vi "Get All.vi"(7 "Q Ref In":refnum<queue>, 8 "error in":errorcluster) -> (0 "error out":errorcluster, 3 "Flushed Elements":T1[](array[typedef]), 5 "Q Ref Out":refnum<queue>)   [LabVIEW 2025, in "Q Wrappers.lvlib"]
uses:
  Q Wrappers.lvlib
  Q Packet.ctl
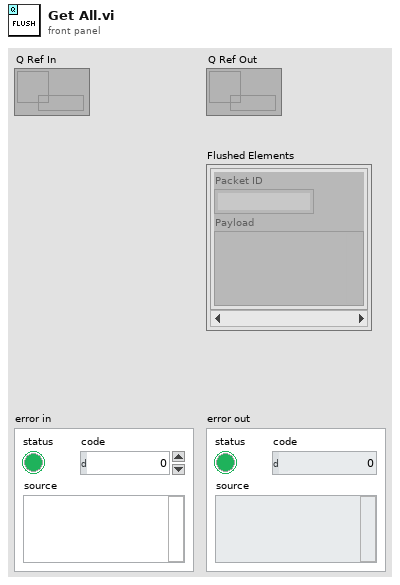
[diagram p1: front panel]
types:
  T1 = typedef "Q Packet.ctl" = cluster{"Packet ID":string, "Payload":variant}
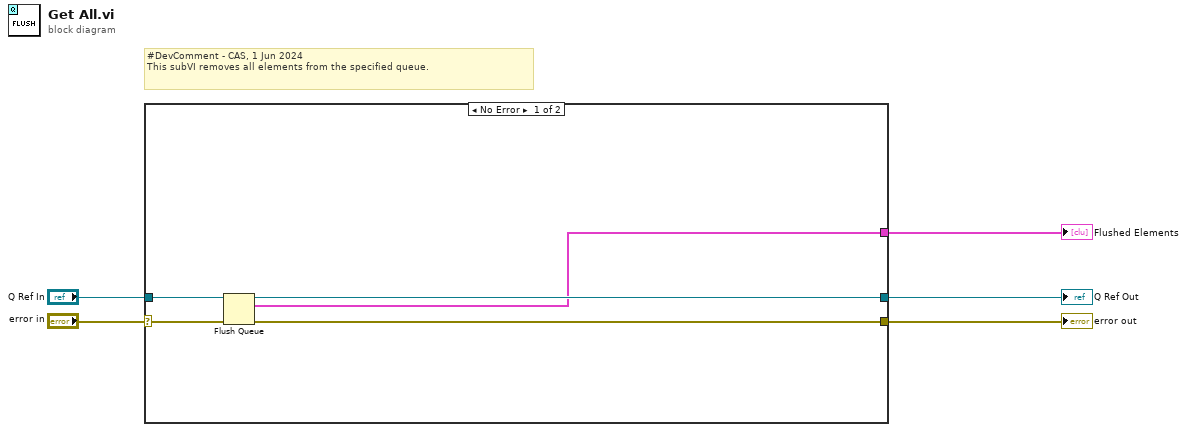
[diagram p0: block diagram]
diagram:
  # "#DevComment - CAS, 1 Jun 2024\nThis subVI removes all elements from the specified queue."
  n1 = case shown="No Error" "error in" {
    selector: "error in" -> [w7 w11]
    tunnel: [w10 w11] -> w4
    tunnel: [w9 _] -> w3
    tunnel: "Q Ref In" -> [w8 _]
    tunnel: [w6 _] -> w1
    frame No Error {
      n2 = Flush Queue(queue=w8, error in (no error)=w7) -> (queue out=w9:refnum<queue>, remaining elements=w6:T1[], error out=w10:errorcluster)
    }
    frame Error {
    }
  }
  "error out" <- w4
  "Q Ref Out" <- w3
  "Flushed Elements" <- w1
